vi "testTCL.vi"   [LabVIEW 2010, in "kevLib2010.lvlib"]
uses:
  kevLib2010.lvlib
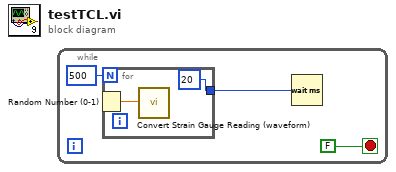
[diagram p0: block diagram]
diagram:
  n1 = while {
    stop <- FALSE stop-if-true
    n2 = for {
      N: 500 -> [_]
      tunnel: [u32 20 ("milliseconds to wait")] -> w1
      n3 = Random Number (0-1)() -> (number: 0 to 1=w5:dbl)
      n4 = call <vilib>:"Convert Strain Gauge Reading (waveform).vi"("Vex (3.33)"=w5) -> ()  [unwired: 9 in, 1 out]
    }
    n5 = Wait (ms)(milliseconds to wait=w1) -> ()  [unwired: 1 out]
  }
